vi "Framework.Get Engine Pointer.vi"(11 "Framework in":refnum<class "Framework.lvclass">) -> (2 "Engine Pointer":refnum<class "Memory.Pointer.lvclass">, 3 "Framework out":refnum<class "Framework.lvclass">)   [LabVIEW 2017, in "DSF Core.lvlib" / "Framework.lvclass"]
uses:
  Framework.lvclass
  <vilib>/NI/Memory Manager/Classes/Pointer/Memory.Pointer.lvclass
  Framework.lvclass/Framework.ctl
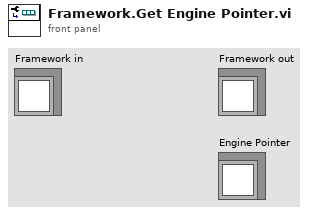
[diagram p1: front panel]
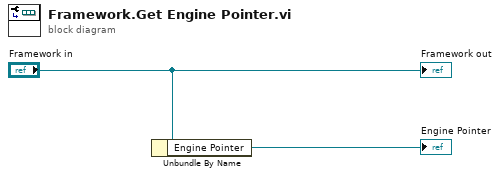
[diagram p0: block diagram]
diagram:
  n1 = Unbundle By Name("Framework in") -> ("Engine Pointer"=→"Engine Pointer":refnum<class "Memory.Pointer.lvclass">)
  "Framework out" <- "Framework in"
